vi "Limit Switch Test.vi"(9 "Progress":string, 10 "ProgressText":string) -> (2 "EndTestText":string)   [LabVIEW 2012]
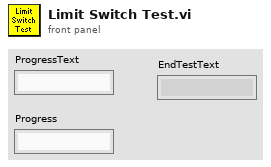
[diagram p1: front panel]
types:
  T1 = typedef "WPI_DigitalInputDevRef.ctl" = cluster{"DevStatus":errorcluster, "DIO Channel":T2, "Digital Module":T3}
  T2 = typedef "FPGA_DIOChannel.ctl" = enum8{"DIO 1", "DIO 2", "DIO 3", "DIO 4", "DIO 5", "DIO 6", "DIO 7", "DIO 8", "DIO 9", "DIO 10", "DIO 11", "DIO 12", "DIO 13", "DIO 14", "Invalid"}
  T3 = typedef "FPGA_TypedefDigitalModule.ctl" = enum16{"Digital Module 1", "Digital Module 2"}
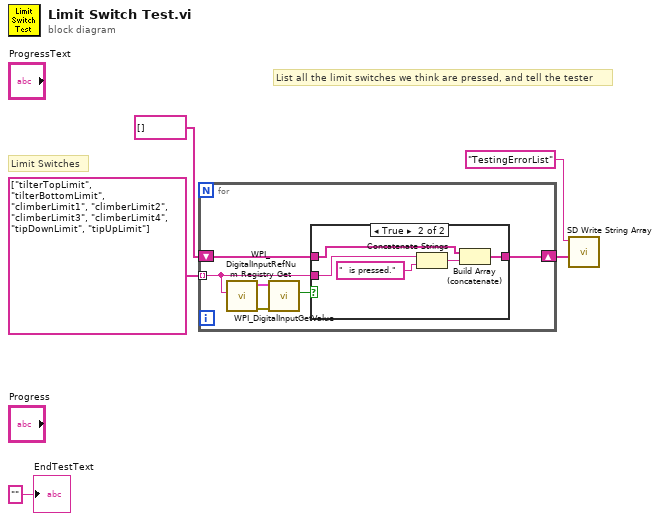
[diagram p0: block diagram]
diagram:
  # "List all the limit switches we think are pressed, and tell the tester"
  # "Limit Switches"
  n1 = for {
    tunnel: string[] ["tilterTopLimit", "tilterBottomLimit", "climberLimit1", "climberLimit2", "climberLimit3", "climberLimit4", "tipDownLimit", "tipUpLimit"] -> [w8] mode=indexing
    shift-right: [w6] -> w4
    shift-left: string[] [] ("String Array") -> [w7]
    n2 = call <vilib>:"WPI_DigitalInputRefNum Registry Get.vi"("refnum name"=w8) -> ("error out"=w11:errorcluster, "DigitalInputDevRef"=w10:T1)  [unwired: 9 in]
    n3 = call <vilib>:"WPI_DigitalInputGetValue.vi"("error in (no error)"=w11, "DigitalInputDevRef"=w10) -> ("Value"=w9:bool)  [unwired: 7 in, 2 out]
    n4 = case shown="True" w9 {
      tunnel: w8 -> [_ w17]
      tunnel: w7 -> [w12 w15]
      tunnel: [w12 w13] -> w6
      frame False {
      }
      frame True {
        n5 = Concatenate Strings(w17, "  is pressed." ("string")) -> (w14:string)
        n6 = Build Array (concatenate)(w15, w14) -> (w13:string[])
      }
    }
  }
  n7 = call <vilib>:"SD Write String Array.vi"("String Array"=w4, "Name"="TestingErrorList") -> ()  [unwired: 8 in, 2 out]
  "EndTestText" <- "" ("EndTestText")
